vi "Untitled 41.vi"() -> ()   [LabVIEW 2017]
panel:
  out "Out":u8 format="%.0x"
  in  "address":string="192.168.10.22"
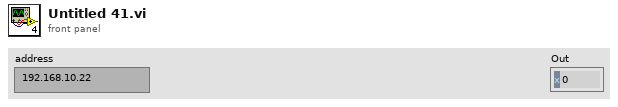
[diagram p1: front panel]
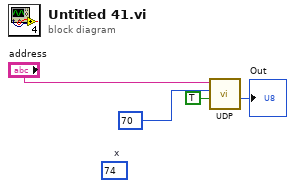
[diagram p0: block diagram]
diagram:
  (unwired) u16 74  # x
  n1 = call "UDP.vi"("Read (TRUE)"=TRUE, "Address"=u32 70, "IP address"="address") -> ("Out"=→"Out":u8)  [unwired: 6 in, 1 out]
